vi "Add Line Feed.vi"(4 "Command string":string) -> (1 "Concatenated string":string)   [LabVIEW 2025, in "Chroma 19572.lvlib"]
uses:
  <instrlib>/Chroma 19572/Chroma 19572.lvlib
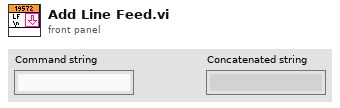
[diagram p1: front panel]
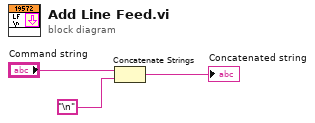
[diagram p0: block diagram]
diagram:
  n1 = Concatenate Strings("Command string", "\n") -> (→"Concatenated string":string)
